vi "Convert Table to Channel Linkages.vi"(8 "error in (no error)":errorcluster, 10 "Item Names":string[][](array[string]), 11 "Item Ref in":T1=18446744073709551615 format="%.0x") -> (0 "error out":errorcluster, 2 "Linkages":T2[](array[typedef]), 3 "Item Ref out":T1 format="%.0x")   [LabVIEW 2019, in "Instrument Addon System Explorer.lvlib"]
uses:
  Instrument Addon System Explorer.lvlib
  Shared/Types/Linked Channel Cluster.ctl
  Shared/Instrument Addon Shared.lvlib
  <vilib>/NI VeriStand/Custom Device API/Custom Device API.lvlib
  NationalInstruments.VeriStand.SystemStorage
  Shared/Constants.vi
  <vilib>/NI VeriStand/Custom Device API/Custom Device Item Ref.ctl
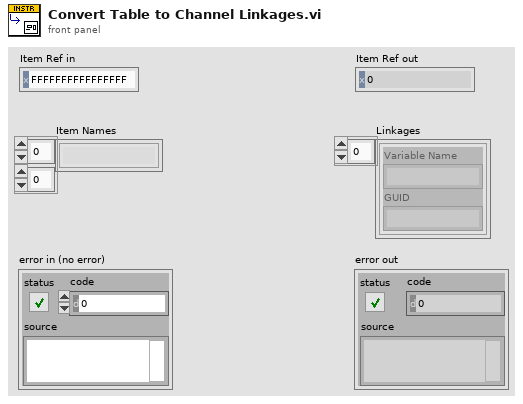
[diagram p1: front panel]
types:
  T1 = typedef "Custom Device API.lvlib/Custom Device Item Ref.ctl" = u64
  T2 = typedef "Instrument Addon Shared.lvlib/Linked Channel Cluster.ctl" = cluster{"Variable Name":string, "GUID":string}
  T3 = typedef "Custom Device API.lvlib/Custom Device Pointer.ctl" = refnum<k24>
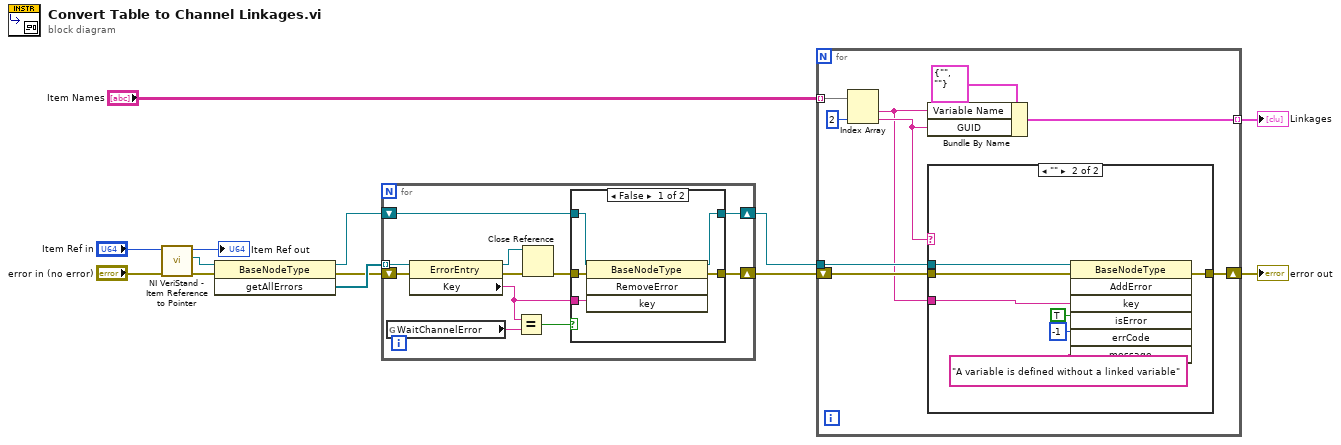
[diagram p0: block diagram]
diagram:
  n1 = call <vilib>:"NI VeriStand - Item Reference to Pointer.vi"("error in (no error)"="error in (no error)", "Item Ref in"="Item Ref in") -> ("error out"=w8:errorcluster, "Node Pointer"=w9:T3, "Item Ref out"=→"Item Ref out":T1)  [unwired: 6 in, 1 out]
  n2 = invoke class="BaseNodeType" method="getAllErrors"(reference=w9, error in=w8) -> (reference out=w2:T3, error out=w4:errorcluster, "getAllErrors"=w5:refnum<k24>[])  [unwired: 1 in]
  n3 = for {
    tunnel: w5 -> [w24] mode=indexing
    shift-right: [w16] -> w3
    shift-left: w4 -> [w22]
    shift-right: [w18] -> w1
    shift-left: w2 -> [w19]
    n4 = global read "Constants.vi" "WaitChannelError"() -> (w23:string)
    n5 = property class="ErrorEntry"(reference=w24, error in=w22) -> (reference out=w21:refnum<k24>, error out=w20:errorcluster, "Key"=w15:string)
    n6 = Equal?(x=w15, y=w23) -> (x = y?=w14:bool)
    n7 = Close Reference(reference=w21, error in (no error)=w20) -> (error out=w17:errorcluster)
    n8 = case shown="False" w14 {
      tunnel: w19 -> [w29 w30]
      tunnel: [w28 w30] -> w18
      tunnel: w17 -> [w27 w31]
      tunnel: [w26 w31] -> w16
      tunnel: w15 -> [w25 _]
      frame False {
        n9 = invoke class="BaseNodeType" method="RemoveError"(reference=w29, error in=w27, "key"=w25) -> (reference out=w28:T3, error out=w26:errorcluster)  [unwired: 1 in, 2 out]
      }
      frame True {
      }
    }
  }
  n10 = for {
    tunnel: "Item Names" -> [w40] mode=indexing
    tunnel: [w37] -> w13 mode=indexing
    tunnel: w1 -> [w34]
    shift-right: [w33] -> w7
    shift-left: w3 -> [w36]
    n11 = Index Array(array=w40, index #2=2 ("index")) -> (element #1=w32:string, element #2=w35:string)  [unwired: 1 in]
    n12 = Bundle By Name(cluster=T2 {"Variable Name"="", "GUID"=""}, "Variable Name"=w32, "GUID"=w35) -> (w37:T2)
    n13 = case shown="\"\"" w35 {
      tunnel: w36 -> [w41 w45]
      tunnel: w34 -> [_ w44]
      tunnel: [w41 w43] -> w33
      tunnel: w32 -> [_ w42]
      frame Default {
      }
      frame "" {
        n14 = invoke class="BaseNodeType" method="AddError"(reference=w44, error in=w45, "key"=w42, "isError"=TRUE, "errCode"=-1, "message"="A variable is defined without a linked variable") -> (error out=w43:errorcluster)  [unwired: 1 in, 6 out]
      }
    }
  }
  "Linkages" <- w13
  "error out" <- w7
